vi "I2S Read(David Documentation).vi"(7 "I2S.WL":u16=32, 8 "I2S.BitCount":u16=31, 9 "I2S.RECDAT IN":bool, 10 "I2S.RECLRC IN":bool, 11 "I2S.BCLK IN":bool) -> (2 "Audio Signals":T1, 3 "Data Channel":bool)   [LabVIEW 2015]
uses:
  Audio Signals.ctl
panel:
  # "Overview: Read digital audio data."
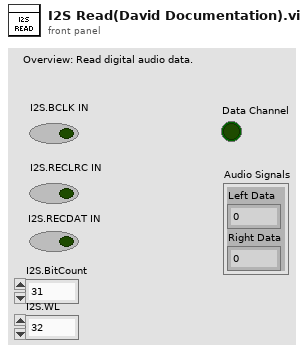
[diagram p1: front panel]
types:
  T1 = typedef "Audio Signals.ctl" = cluster{"Left Data":u32, "Right Data":u32}
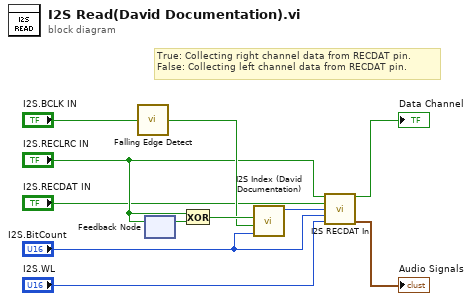
[diagram p0: block diagram]
diagram:
  # "True: Collecting right channel data from RECDAT pin.\nFalse: Collecting left channel data from RECDAT pin."
  n1 = call "Falling Edge Detect.vi"("Signal"="I2S.BCLK IN") -> ("Trigger?"=w8:bool)
  n2 = feedback #1() -> (w10:bool)  [unwired: 1 in]
  n3 = feedback-in #1("I2S.RECLRC IN") -> ()
  n4 = Exclusive Or(1:w10, 2:"I2S.RECLRC IN") -> (0:w9:bool)
  n5 = call "I2S Index (David Documentation).vi"("Bit Count"="I2S.BitCount", "Update"=w8, "Change Channel"=w9) -> ("Value Out"=w5:u16)  [unwired: 8 in]
  n6 = call "I2S RECDAT In.vi"("I2S.RECLRC IN"="I2S.RECLRC IN", "I2S.RECDAT IN"="I2S.RECDAT IN", "Data Index"=w5, "Bit Count"="I2S.BitCount", "Word Length"="I2S.WL") -> ("Data Channel"=→"Data Channel":bool, "Audio Signals"=→"Audio Signals":T1)  [unwired: 9 in]
